vi "Instances check dates.vi"(6 "Array in":string[](array[string]), 7 "Year":i32, 8 "Month":i32, 10 "Dates undelivered":timestamp[](array[timestamp])) -> (3 "Dates undelivered out":timestamp[](array[timestamp]))   [LabVIEW 2015]
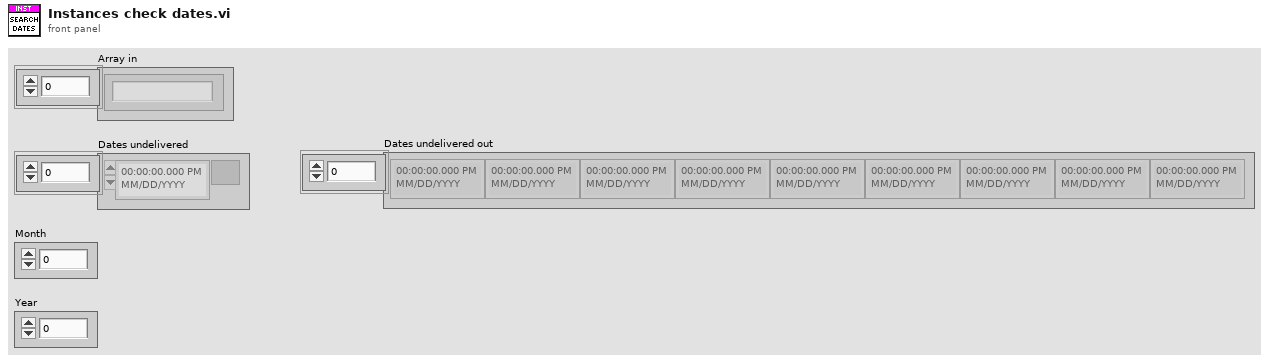
[diagram p1: front panel]
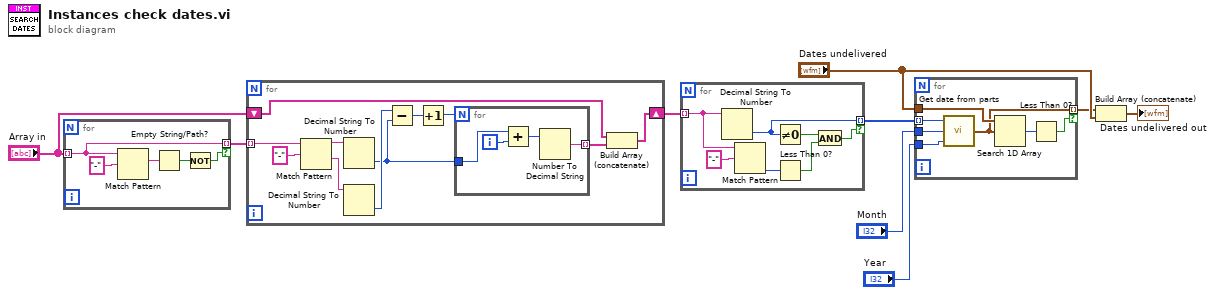
[diagram p0: block diagram]
diagram:
  n1 = for {
    tunnel: "Array in" -> [w10] mode=indexing
    tunnel: [w10] -> w5 mode=indexing if=w11
    n2 = Match Pattern(string=w10, regular expression="-") -> (match substring=w13:string)  [unwired: 1 in, 3 out]
    n3 = Empty String/Path?(string/path=w13) -> (empty?=w12:bool)
    n4 = Not(x=w12) -> (.not. x?=w11:bool)
  }
  n5 = for {
    tunnel: w5 -> [w25] mode=indexing
    shift-right: [w15] -> w7
    shift-left: "Array in" -> [w17]
    n6 = Match Pattern(string=w25, regular expression="-") -> (before substring=w23:string, after substring=w22:string)  [unwired: 1 in, 2 out]
    n7 = Decimal String To Number(string=w23) -> (number=w18:i32)  [unwired: 2 in, 1 out]
    n8 = Decimal String To Number(string=w22) -> (number=w21:i32)  [unwired: 2 in, 1 out]
    n9 = Subtract(x=w21, y=w18) -> (x-y=w20:i32)
    n10 = Increment(x=w20) -> (x+1=w19:i32)
    n11 = for {
      N: w19 -> [_]
      tunnel: w18 -> [w28]
      tunnel: [w26] -> w16 mode=indexing
      i -> [w29]
      n12 = Add(x=w28, y=w29) -> (x+y=w27:i32)
      n13 = Number To Decimal String(number=w27) -> (decimal integer string=w26:string)  [unwired: 1 in]
    }
    n14 = Build Array (concatenate)(w17, w16) -> (w15:string[])
  }
  n15 = for {
    tunnel: w7 -> [w35] mode=indexing
    tunnel: [w36] -> w1 mode=indexing if=w30
    n16 = Decimal String To Number(string=w35) -> (number=w36:i32)  [unwired: 2 in, 1 out]
    n17 = Match Pattern(string=w35, regular expression="-") -> (offset past match=w33:i32)  [unwired: 1 in, 3 out]
    n18 = Not Equal To 0?(x=w36) -> (x != 0?=w31:bool)
    n19 = Less Than 0?(x=w33) -> (x < 0?=w32:bool)
    n20 = And(x=w31, y=w32) -> (x .and. y?=w30:bool)
  }
  n21 = for {
    tunnel: w1 -> [w43] mode=indexing
    tunnel: "Dates undelivered" -> [w42]
    tunnel: [w40] -> w2 mode=indexing if=w39
    tunnel: "Month" -> [w38]
    tunnel: "Year" -> [w37]
    n22 = call "Get date from parts.vi"("Year"=w37, "Month"=w38, "Date"=w43) -> ("Date Stamp"=w40:timestamp)
    n23 = Search 1D Array(1D array=w42, element=w40) -> (index of element=w41:i32)  [unwired: 1 in]
    n24 = Less Than 0?(x=w41) -> (x < 0?=w39:bool)
  }
  n25 = Build Array (concatenate)(w2, "Dates undelivered") -> (→"Dates undelivered out":timestamp[])
